vi "Untitled 1.vi"() -> ()   [LabVIEW 2019]
uses:
  <vilib>/FPGAPlugInAG/myRIO-1900/niLvFpga_Open_myRIO-1900.vi
  <vilib>/rvi/interface/common/dynamic/niFpgaDynamicAddResources.vi
  <vilib>/Utility/error.llb/Error Cluster From Error Code.vi
  <vilib>/rvi/errors/niLvFpgaAdjustHostInterfaceError.vi
  <vilib>/rvi/interface/nirviOpenFPGA/nirviOpenFPGA.xnode
  UntitledProject1_FPGATarget_FPGAMainDefault_WVuur2APCNE.lvbitx
  <vilib>/rvi/interface/nirviReadWriteControl/nirviReadWriteControl.xnode
  <vilib>/rvi/interface/Simulation/niFpgaSimulationCallBeginRW.vi
  NiFpgaLv.dll
panel:
  out "Ping.A.State":bool
  out "Ping.A.Tick":u32
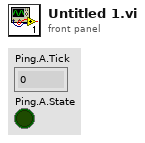
[diagram p1: front panel]
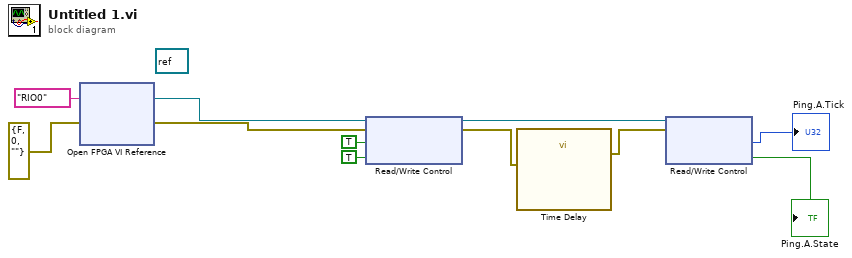
[diagram p0: block diagram]
diagram:
  (unwired) refnum<k20> refnum ("Type")
  n1 = xnode "Open FPGA VI Reference"("error in"=errorcluster {"status"=FALSE, "code"=0, "source"=""}, "resource name"=tag "RIO0") -> ("FPGA VI Reference Out"=w3:refnum<k20>, "error out"=w10:errorcluster)
  n2 = xnode "Read/Write Control"("FPGA VI Reference In"=w3, "error in"=w10, "Ping.A.enable"=TRUE, "Ping.A.Start"=TRUE) -> ("FPGA VI Reference Out"=w6:refnum<k20>, "error out"=w8:errorcluster)
  n3 = call "Time Delay"("error in (no error)"=w8) -> ("error out"=w7:errorcluster)  [unwired: 10 in]
  n4 = xnode "Read/Write Control"("FPGA VI Reference In"=w6, "error in"=w7) -> ("Ping.A.Tick"=→"Ping.A.Tick":u32, "Ping.A.State"=→"Ping.A.State":bool)  [unwired: 2 out]
